vi "Sample Transfer Check Samples.vi"(8 "error in (no error)":errorcluster, 11 "cRIO-CO2 in":refnum<class "cRIO-CO2.lvclass">) -> (0 "error out":errorcluster, 1 "Target not Empty":bool, 2 "Same Sample in Source and Target":bool, 3 "cRIO-CO2 out":refnum<class "cRIO-CO2.lvclass">, 5 "Same Sample AND Target not Empty":bool)   [LabVIEW 2015, in "cRIO-Carbondioxide.lvlib" / "cRIO-CO2.lvlib" / "cRIO-CO2.lvclass"]
uses:
  cRIO-CO2.lvclass
  cRIO-CO2.lvclass/cRIO-CO2.ctl
  subs/Sample/Sample.lvclass/Sample.ctl
  subs/Sample/Sample.lvclass
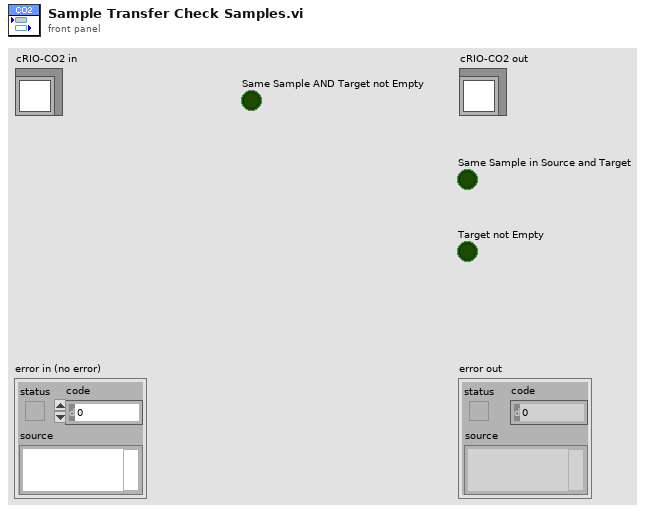
[diagram p1: front panel]
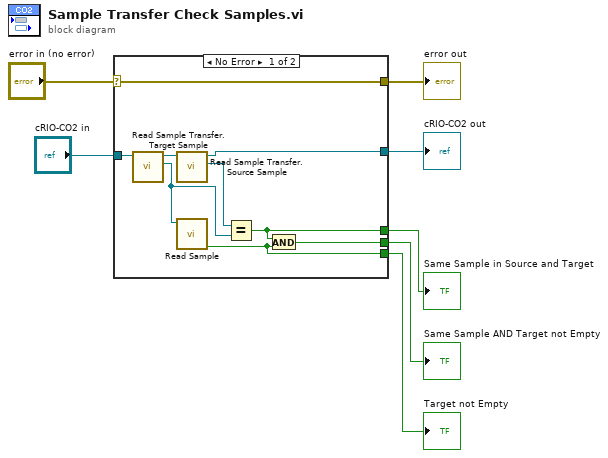
[diagram p0: block diagram]
diagram:
  n1 = case shown="No Error" "error in (no error)" {
    selector: "error in (no error)" -> [w16 w18]
    tunnel: [w16 w18] -> w6
    tunnel: [w13 w17] -> w4
    tunnel: "cRIO-CO2 in" -> [w15 w17]
    tunnel: [w11 _] -> w3
    tunnel: [w10 _] -> w2
    tunnel: [w9 _] -> w1
    frame No Error {
      n2 = call "Read Sample Transfer.Target Sample.vi"("cRIO-CO2 in"=w15) -> ("Sample.lvclass"=w12:refnum<class "Sample.lvclass">, "cRIO-CO2 out"=w14:refnum<class "cRIO-CO2.lvclass">)  [unwired: 9 in]
      n3 = call "Read Sample Transfer.Source Sample.vi"("cRIO-CO2 in"=w14) -> ("Sample.lvclass"=w8:refnum<class "Sample.lvclass">, "cRIO-CO2 out"=w13:refnum<class "cRIO-CO2.lvclass">)  [unwired: 9 in]
      n4 = call "Read Sample.vi"("Sample in"=w12) -> ("Sample In"=w10:bool)  [unwired: 6 in, 4 out]
      n5 = Equal?(x=w8, y=w12) -> (x = y?=w11:bool)
      n6 = And(x=w11, y=w10) -> (x .and. y?=w9:bool)
    }
    frame Error {
    }
  }
  "error out" <- w6
  "cRIO-CO2 out" <- w4
  "Same Sample in Source and Target" <- w3
  "Target not Empty" <- w2
  "Same Sample AND Target not Empty" <- w1
